vi "Broadcast Data Msg.vi"(7 "Message Priority (Normal)":T1=enum."Normal", 8 "error in (no error)":errorcluster, 10 "Concrete Data Msgs":refnum<class "Data Msg.lvclass">[](array[class]), 11 "Broadcast Registry In":refnum<class "Broadcast Registry.lvclass">) -> (0 "error out":errorcluster, 3 "Broadcast Registry Out":refnum<class "Broadcast Registry.lvclass">)   [LabVIEW 2016, in "Data Broadcasting.lvlib" / "Broadcast Registry.lvclass"]
doc: "Broadcasts a data message to all registered Listeners. Each Listener receives its own <b>Concrete Data Msg</b>. The private data element(s) should be written to each data msg prior to broadcasting.\n\n-------------\nCopyright (c) 2013, Staab Engineering, a Texas Limited Liability Company\nAll rights reserved.\n\nRedistribution and use in source and binary forms, with or without modification, are permitted provided that the following conditions are met:\n\n1. Redistributions of source code must retain the above copyright notice, this list of conditions and the following disclaimer.\n2. Redistributions in binary form must reproduce the above copyright notice, this list of conditions and the following disclaimer in the documentation and/or other materials provided with the distribution.\n\nTHIS SOFTWARE IS PROVIDED BY THE COPYRIGHT HOLDERS AND CONTRIBUTORS \"AS IS\" AND ANY EXPRESS OR IMPLIED WARRANTIES, INCLUDING, BUT NOT LIMITED TO, THE IMPLIED WARRANTIES OF MERCHANTABILITY AND FITNESS FOR A PARTICULAR PURPOSE ARE DISCLAIMED. IN NO EVENT SHALL THE COPYRIGHT HOLDER OR CONTRIBUTORS BE LIABLE FOR ANY DIRECT, INDIRECT, INCIDENTAL, SPECIAL, EXEMPLARY, OR CONSEQUENTIAL DAMAGES (INCLUDING, BUT NOT LIMITED TO, PROCUREMENT OF SUBSTITUTE GOODS OR SERVICES; LOSS OF USE, DATA, OR PROFITS; OR BUSINESS INTERRUPTION) HOWEVER CAUSED AND ON ANY THEORY OF LIABILITY, WHETHER IN CONTRACT, STRICT LIABILITY, OR TORT (INCLUDING NEGLIGENCE OR OTHERWISE) ARISING IN ANY WAY OUT OF THE USE OF THIS SOFTWARE, EVEN IF ADVISED OF THE POSSIBILITY OF SUCH DAMAGE."
uses:
  <userlib>/_Frameworks/Staab/AF Data Broadcasting/Data Broadcasting/Broadcast Registry/Broadcast Registry.lvclass
  <userlib>/_Frameworks/Staab/AF Data Broadcasting/Data Broadcasting/Data Msg/Data Msg.lvclass
  C:/Program Files (x86)/National Instruments/LabVIEW 2016/vi.lib/ActorFramework/Message/Message.lvclass
  <vilib>/ActorFramework/Message Enqueuer/Message Priority.ctl
  <userlib>/_Frameworks/Staab/AF Data Broadcasting/Data Broadcasting/Broadcast Registry/Broadcast Registry.lvclass/Broadcast Registry.ctl
  <vilib>/ActorFramework/Message Enqueuer/Message Enqueuer.lvclass/Message Enqueuer.ctl
  <vilib>/ActorFramework/Message Priority Queue/Priority Enqueue.vi
  <vilib>/ActorFramework/Message Enqueuer/Message Enqueuer.lvclass
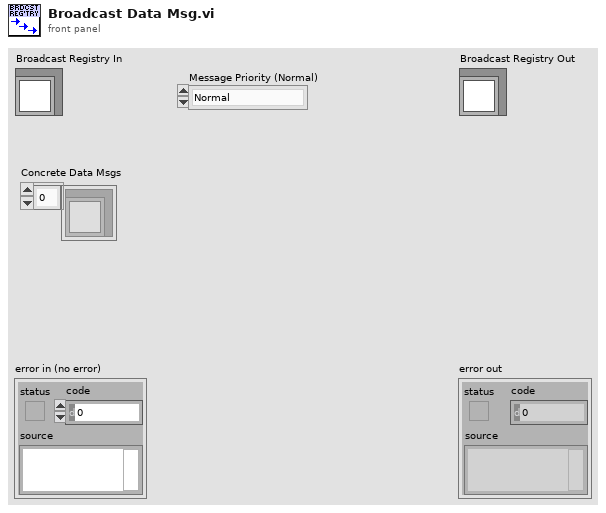
[diagram p1: front panel]
types:
  T1 = typedef "Actor Framework.lvlib/Message Enqueuer.lvclass/Message Priority.ctl" = enum16{"Low", "Normal", "High"}
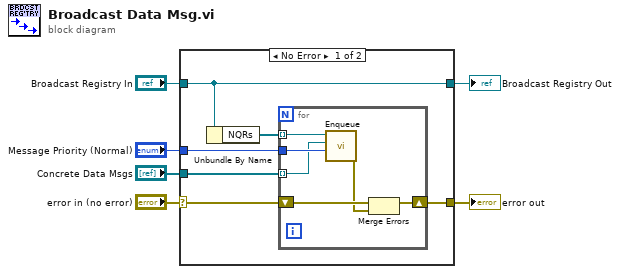
[diagram p0: block diagram]
diagram:
  n1 = case shown="No Error" "error in (no error)" {
    selector: "error in (no error)" -> [w8 w19]
    tunnel: "Broadcast Registry In" -> [w11 w20]
    tunnel: [w11 w20] -> w5
    tunnel: [w7 w19] -> w4
    tunnel: "Concrete Data Msgs" -> [w10 _]
    tunnel: "Message Priority (Normal)" -> [w9 _]
    frame No Error {
      n2 = Unbundle By Name(w11) -> ("NQRs"=w12:refnum<class "Message Enqueuer.lvclass">[])
      n3 = for {
        tunnel: w12 -> [w18] mode=indexing
        tunnel: w10 -> [w16] mode=indexing
        tunnel: w9 -> [w17]
        shift-right: [w13] -> w7
        shift-left: w8 -> [w15]
        n4 = call <vilib>:"Enqueue.vi"("Message Priority (Normal)"=w17, "Message"=w16, "Message Enqueuer in"=w18) -> ("error out"=w14:errorcluster)  [unwired: 7 in, 1 out]
        n5 = Merge Errors(w15, w14) -> (w13:errorcluster)
      }
    }
    frame Error {
    }
  }
  "error out" <- w4
  "Broadcast Registry Out" <- w5
